vi "ControlMatrixDialog.vi"() -> (3 "Controllers out":T2)   [LabVIEW 2018]
uses:
  controls/Controller.ctl
  Real-Time/Control Algorithm/Control Algorithm Selection.ctl
panel:
  in  "W2 compensator matrix":T1
  out "Controlador":enum16{"LQG-LTR", "Hinf"}(ring)
  in  "W1 compensator matrix":T1
  in  "Robust controller matrix":T1
  in  "ok":bool caption="Blank"
  out "Singular Values Plot":cluster{"W":dbl[], "Magnitude":dbl[]}[](graph)
  in  "Load Controller matrix":bool caption="Open"
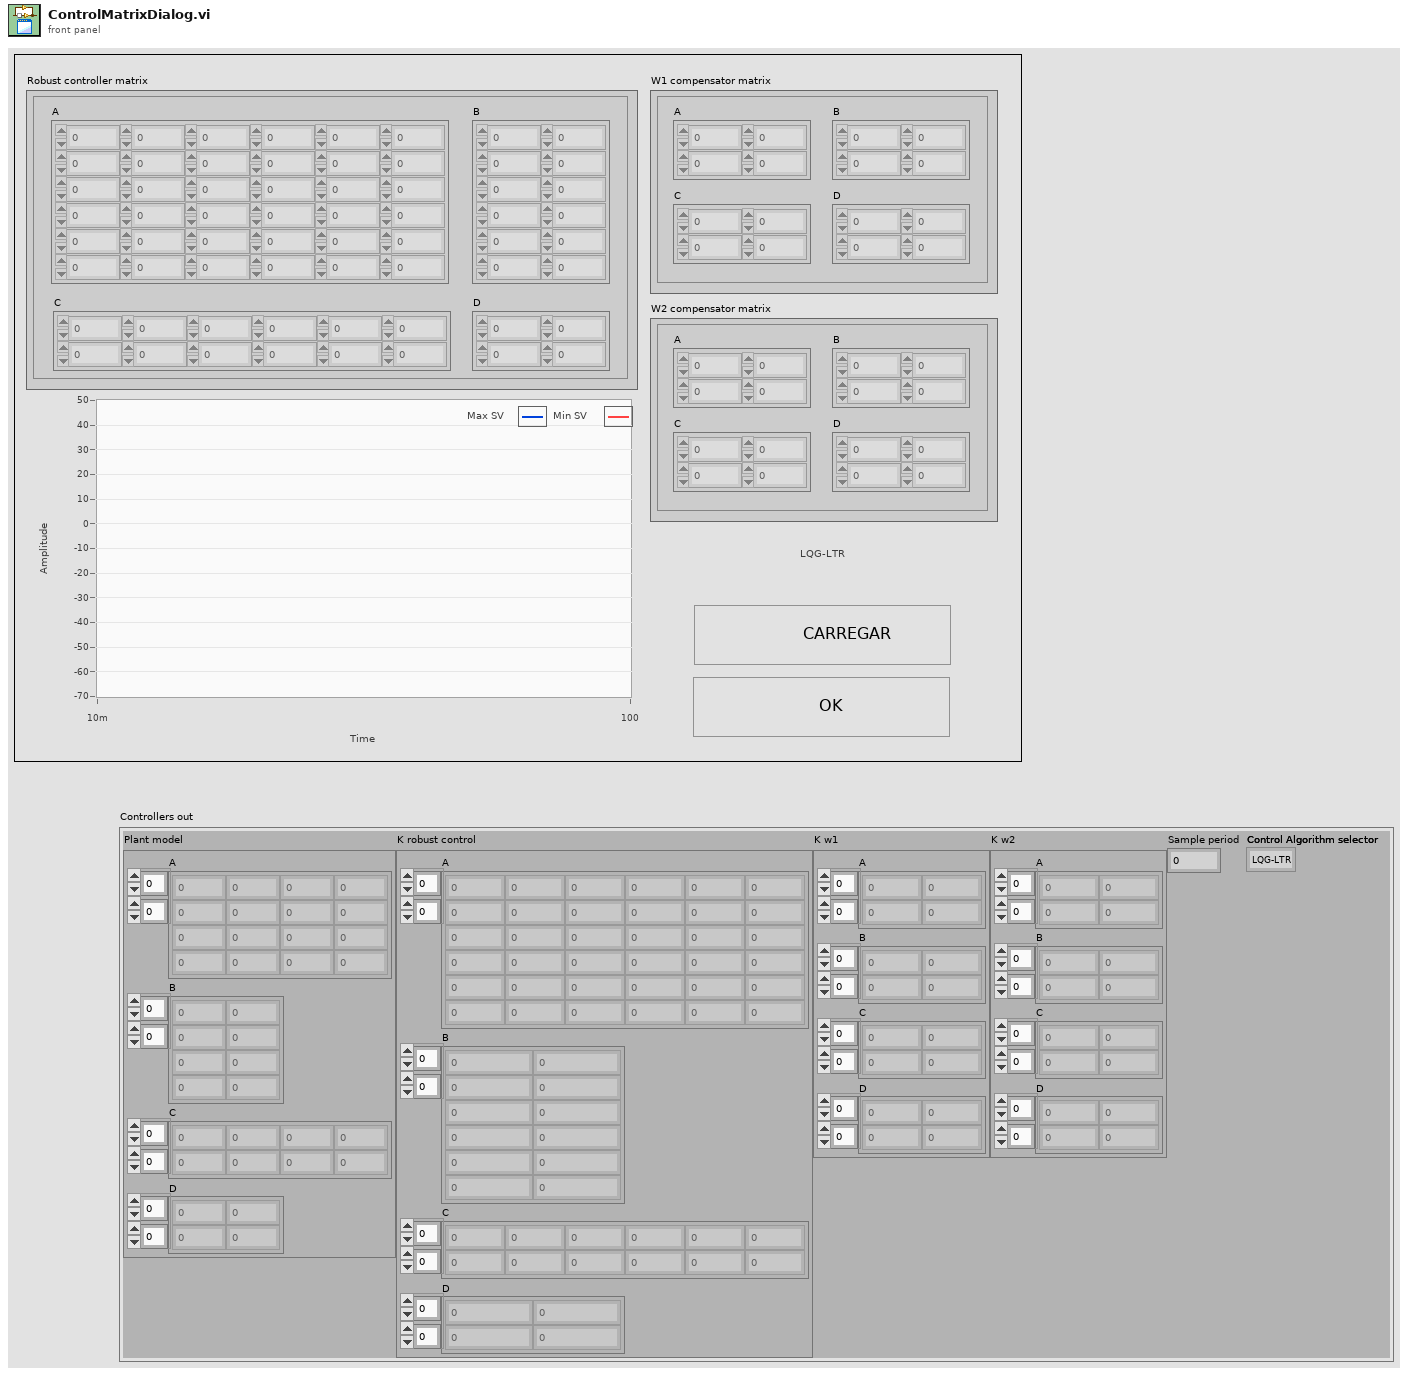
[diagram p1: front panel]
types:
  T1 = cluster{"A":dbl[][], "B":dbl[][], "C":dbl[][], "D":dbl[][]}
  T2 = typedef "Controller.ctl" = cluster{"Plant model":cluster{"A":dbl[][], "B":dbl[][], "C":dbl[][], "D":dbl[][]}, "K robust control":cluster{"A":dbl[][], "B":dbl[][], "C":dbl[][], "D":dbl[][]}, "K w1":cluster{"A":dbl[][], "B":dbl[][], "C":dbl[][], "D":dbl[][]}, "K w2":cluster{"A":dbl[][], "B":dbl[][], "C":dbl[][], "D":dbl[][]}, "Sample period":dbl, "Control Algorithm selector":T3}
  T3 = typedef "Control Algorithm Selection.ctl" = enum16{"LQG-LTR", "Hinf"}
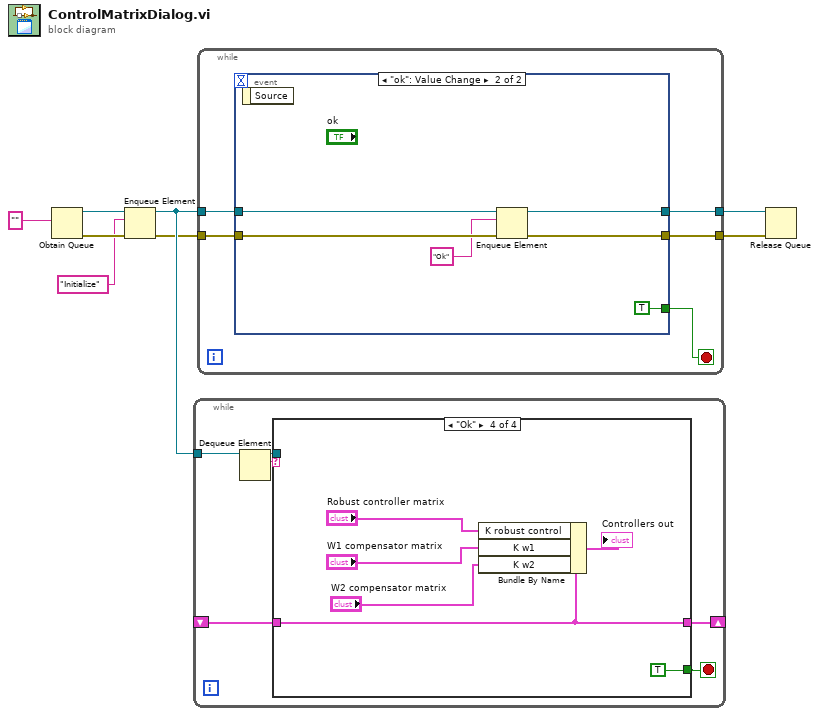
[diagram p0: block diagram]
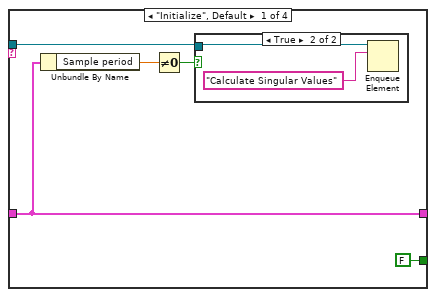
[diagram p2: hidden frame]
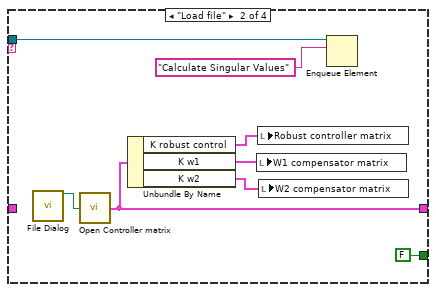
[diagram p4: hidden frame]
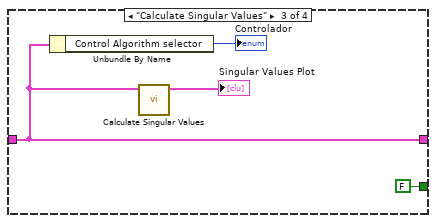
[diagram p5: hidden frame]
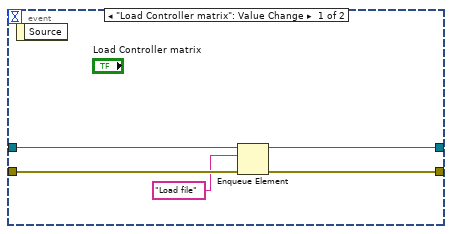
[diagram p6: hidden frame]
diagram:
  n1 = Obtain Queue(element data type="" ("element")) -> (queue out=w6:refnum<queue>, error out=w4:errorcluster)  [unwired: 4 in, 1 out]
  n2 = Enqueue Element(queue=w6, element="Initialize", error in (no error)=w4) -> (queue out=w5:refnum<queue>, error out=w3:errorcluster)  [unwired: 1 in, 1 out]
  n3 = while {
    tunnel: w5 -> [w14]
    shift-right: [w11] -> _
    shift-left: _ -> [w12]
    stop <- w9 stop-if-true
    n4 = Dequeue Element(queue=w14) -> (queue out=w10:refnum<queue>, element=w13:string)  [unwired: 2 in, 2 out]
    n5 = case shown="\"Ok\"" w13 {
      tunnel: w12 -> [w16 _ w30 w36]
      tunnel: [w16 w25 w30 w36] -> w11
      tunnel: w10 -> [w18 w27 _ _]
      tunnel: [FALSE FALSE FALSE TRUE] -> w9
      frame "Initialize", Default {
        n6 = Unbundle By Name(w16) -> ("Sample period"=w19:dbl)
        n7 = Not Equal To 0?(x=w19) -> (x != 0?=w17:bool)
        n8 = case shown="True" w17 {
          tunnel: w18 -> [_ w20]
          frame False {
          }
          frame True {
            n9 = Enqueue Element(queue=w20, element="Calculate Singular Values") -> ()  [unwired: 2 in, 3 out]
          }
        }
      }
      frame "Load file" {
        n10 = call "File Dialog"() -> ("selected path"=w29:path)  [unwired: 12 in, 3 out]
        n11 = call "Open Controller matrix.vi"("file path (dialog if empty)"=w29) -> ("Cluster"=w25:T2)
        n12 = Unbundle By Name(w25) -> ("K robust control"=w22:T1, "K w1"=w24:T1, "K w2"=w23:T1)
        n13 = local write "W1 compensator matrix"(w24) -> ()
        n14 = local write "Robust controller matrix"(w22) -> ()
        n15 = local write "W2 compensator matrix"(w23) -> ()
        n16 = Enqueue Element(queue=w27, element="Calculate Singular Values") -> ()  [unwired: 2 in, 3 out]
      }
      frame "Calculate Singular Values" {
        n17 = Unbundle By Name(w30) -> ("Control Algorithm selector"=→"Controlador":T3)
        n18 = call "Calculate Singular Values.vi"("Controllers in"=w30) -> ("Singular Values Plot"=→"Singular Values Plot":cluster{"W":dbl[], "Magnitude":dbl[]}[])  [unwired: 10 in]
      }
      frame "Ok" {
        n19 = Bundle By Name(cluster=w36, "K robust control"="Robust controller matrix", "K w1"="W1 compensator matrix", "K w2"="W2 compensator matrix") -> (→"Controllers out":T2)
      }
    }
  }
  n20 = while {
    tunnel: w5 -> [w44]
    tunnel: [w43] -> w8
    tunnel: w3 -> [w42]
    tunnel: [w41] -> w7
    stop <- w40 stop-if-true
    n21 = event shown="[1] \"ok\": Value Change" {
      selector: _ -> [_ _]
      dyn-events: _ -> [_ _]
      timeout: _ -> [_ _]
      tunnel: w44 -> [w49 w55]
      tunnel: [w48 w54] -> w43
      tunnel: w42 -> [w47 w53]
      tunnel: [w46 w52] -> w41
      tunnel: [_ TRUE] -> w40
      event "Load Controller matrix": Value Change {
        n22 = event-data() -> ()  [unwired: 1 in, 1 out]
        n23 = Enqueue Element(queue=w49, element="Load file", error in (no error)=w47) -> (queue out=w48:refnum<queue>, error out=w46:errorcluster)  [unwired: 1 in, 1 out]
      }
      event "ok": Value Change {
        n24 = event-data() -> ()  [unwired: 1 in, 1 out]
        n25 = Enqueue Element(queue=w55, element="Ok", error in (no error)=w53) -> (queue out=w54:refnum<queue>, error out=w52:errorcluster)  [unwired: 1 in, 1 out]
      }
    }
  }
  n26 = Release Queue(queue=w8, error in (no error)=w7) -> ()  [unwired: 1 in, 3 out]
